vi "CCE RRMA T030 SubVI02.vi"(9 "sig":i32, 10 "T":i32, 11 "capa":u8[][](array[numeric])) -> (1 "capa u8":u8[][](array[numeric]), 2 "new picture":picture, 3 "imagen suavizada":u32[][](array[numeric]))   [LabVIEW 2020]
doc: "Ceballos Conde Emanuel Rodríguez Ramírez Miguel Ángel 4MV6 Sistemas de visión artificial 2022/1\neste vi permite obtener el suavisado de una imagen teniendo como entrada un arreglo que representa dicha imagen y lo valores T y sig que se utilizan para el metodo de suavisado basado en la campana de Gauss"
panel:
  out "h":dbl[][](array[numeric])
  # "Ceballos Conde Emanuel\nRodríguez Ramírez Miguel Ángel\n4MV6\nSistemas de visión artificial\n2022/1"
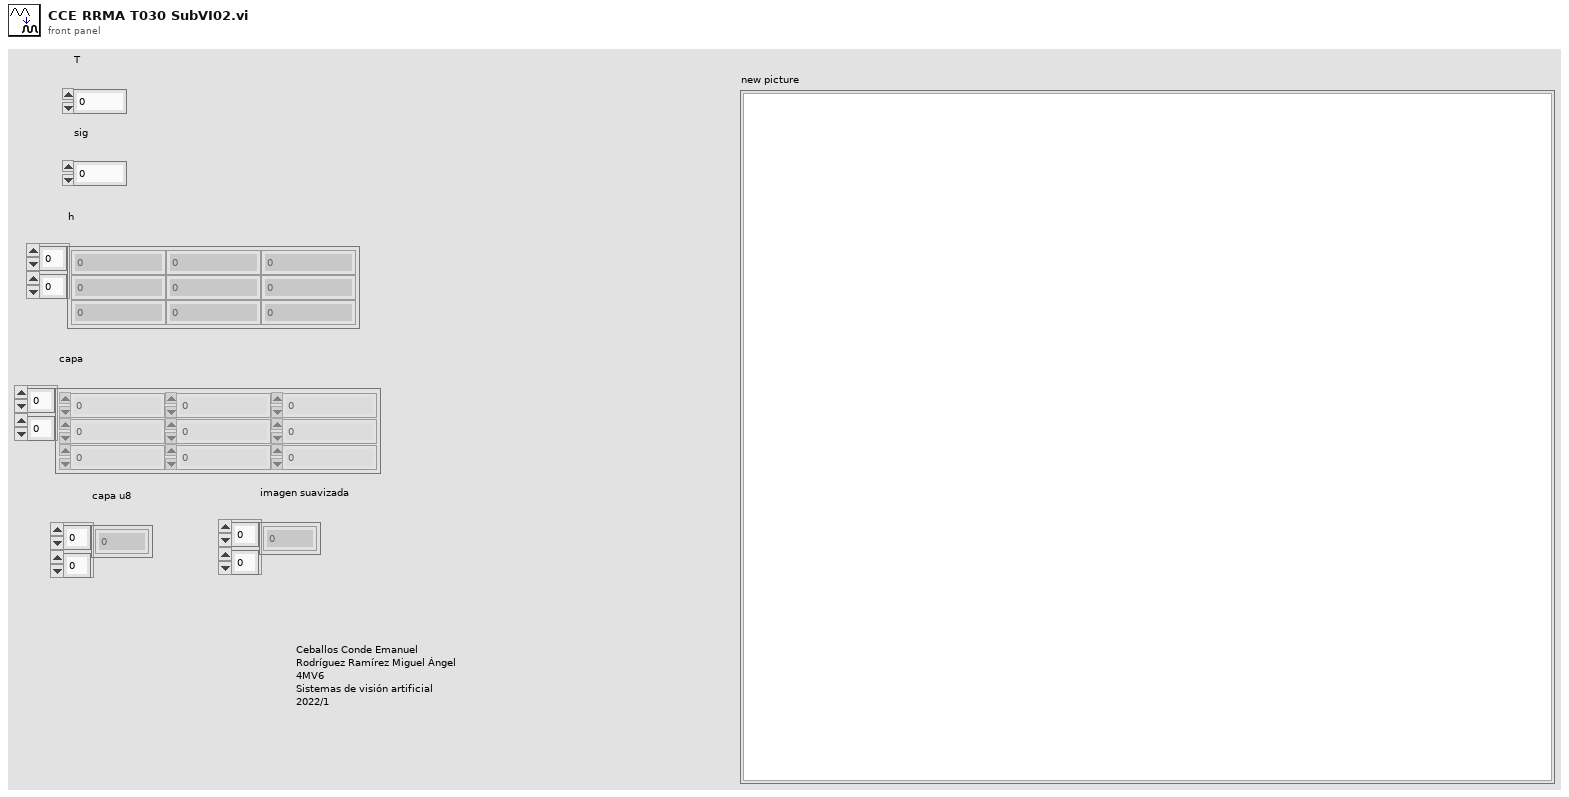
[diagram p1: front panel]
types:
  T1 = typedef "imagedata.ctl" = cluster{"image type":i32, "image depth":i32, "image":u8[], "mask":u8[], "colors":u32[], "Rectangle":cluster{"left":i16, "top":i16, "right":i16, "bottom":i16}}
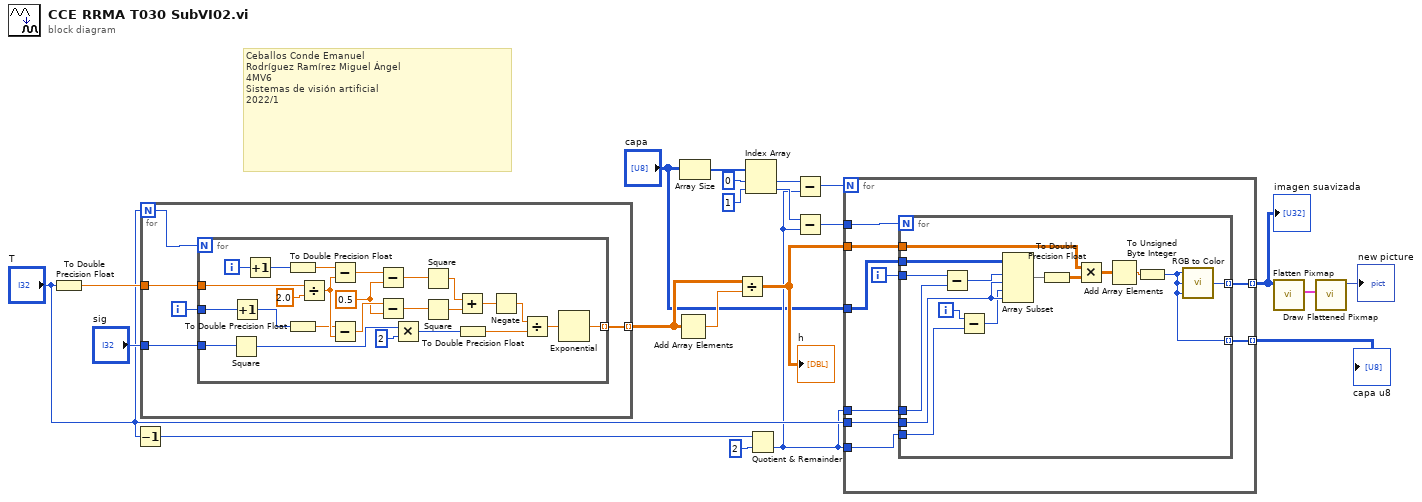
[diagram p0: block diagram]
diagram:
  # "Ceballos Conde Emanuel\nRodríguez Ramírez Miguel Ángel\n4MV6\nSistemas de visión artificial\n2022/1"
  n1 = To Double Precision Float(number="T") -> (double precision float=w18:dbl)
  n2 = Decrement(x="T") -> (x-1=w9:i32)
  n3 = for {
    N: "T" -> [w26]
    tunnel: "sig" -> [w25]
    tunnel: [w24] -> w20 mode=indexing
    tunnel: w18 -> [w23]
    i -> [w22]
    n4 = for {
      N: w26 -> [_]
      tunnel: w25 -> [w51]
      tunnel: [w48] -> w24 mode=indexing
      tunnel: w23 -> [w46]
      tunnel: w22 -> [w41]
      i -> [w35]
      w36 = 0.5 ("y")
      n5 = Square(x=w51) -> (x^2=w30:i32)
      n6 = Increment(x=w41) -> (x+1=w33:i32)
      n7 = Increment(x=w35) -> (x+1=w34:i32)
      n8 = To Double Precision Float(number=w34) -> (double precision float=w29:dbl)
      n9 = To Double Precision Float(number=w33) -> (double precision float=w28:dbl)
      n10 = Divide(x=w46, y=2.0) -> (x/y=w37:dbl)
      n11 = Subtract(x=w29, y=w37) -> (x-y=w47:dbl)
      n12 = Subtract(x=w28, y=w37) -> (x-y=w43:dbl)
      n13 = Subtract(x=w47, y=w36) -> (x-y=w44:dbl)
      n14 = Subtract(x=w43, y=w36) -> (x-y=w42:dbl)
      n15 = Multiply(x=w30, y=2) -> (x*y=w49:i32)
      n16 = Square(x=w44) -> (x^2=w40:dbl)
      n17 = Square(x=w42) -> (x^2=w39:dbl)
      n18 = Add(x=w40, y=w39) -> (x+y=w38:dbl)
      n19 = To Double Precision Float(number=w49) -> (double precision float=w27:dbl)
      n20 = Negate(x=w38) -> (-x=w31:dbl)
      n21 = Divide(x=w31, y=w27) -> (x/y=w32:dbl)
      n22 = Exponential(1:w32) -> (0:w48:dbl)
    }
  }
  n23 = Add Array Elements(numeric array=w20) -> (sum=w19:dbl)
  n24 = Array Size(array="capa") -> (size(s)=w17:i32[])
  n25 = Divide(x=w20, y=w19) -> (x/y=w14:dbl[][])
  "h" <- w14
  n26 = Index Array(array=w17, index #1=0 ("index"), index #2=1 ("index")) -> (element #1=w7:i32, element #2=w4:i32)
  n27 = Quotient & Remainder(x=w9, y=2) -> (floor(x/y)=w3:i32)  [unwired: 1 out]
  n28 = Subtract(x=w7, y=w3) -> (x-y=w6:i32)
  n29 = Subtract(x=w4, y=w3) -> (x-y=w5:i32)
  n30 = for {
    N: w6 -> [_]
    tunnel: w14 -> [w60]
    tunnel: "capa" -> [w59]
    tunnel: [w58] -> w13 mode=indexing
    tunnel: "T" -> [w57]
    tunnel: w5 -> [w56]
    tunnel: w3 -> [w54]
    tunnel: w3 -> [w53]
    tunnel: [w52] -> w1 mode=indexing
    i -> [w55]
    n31 = for {
      N: w56 -> [_]
      tunnel: w60 -> [w75]
      tunnel: w59 -> [w74]
      tunnel: [w70] -> w58 mode=indexing
      tunnel: w57 -> [w72]
      tunnel: w55 -> [w66]
      tunnel: w54 -> [w65]
      tunnel: w53 -> [w62]
      tunnel: [w61] -> w52 mode=indexing
      i -> [w63]
      n32 = Subtract(x=w66, y=w65) -> (x-y=w67:i32)
      n33 = Subtract(x=w63, y=w62) -> (x-y=w64:i32)
      n34 = Array Subset(array=w74, index (row)=w67, length (row)=w72, index (col)=w64, length (col)=w72) -> (w68:u8[][])
      n35 = To Double Precision Float(number=w68) -> (double precision float=w69:dbl[][])
      n36 = Multiply(x=w75, y=w69) -> (x*y=w73:dbl[][])
      n37 = Add Array Elements(numeric array=w73) -> (sum=w71:dbl)
      n38 = To Unsigned Byte Integer(number=w71) -> (unsigned 8bit integer=w61:u8)
      n39 = call <vilib>:"RGB to Color.vi"("B"=w61, "G"=w61, "R"=w61) -> ("Color"=w70:u32)
    }
  }
  "imagen suavizada" <- w13
  "capa u8" <- w1
  n40 = call <vilib>:"Flatten Pixmap.vi"("24-bit pixmap"=w13) -> ("image data"=w12:T1)  [unwired: 10 in]
  n41 = call <vilib>:"Draw Flattened Pixmap.vi"("image data"=w12) -> ("new picture"=→"new picture":picture)  [unwired: 8 in]
